vi "Primer programa1.vi"() -> ()   [LabVIEW 2020]
panel:
  out "String":string
  out "Resultado":dbl
  in  "y":dbl
  in  "x":dbl
  in  "Opcion":string(combo)="Suma"
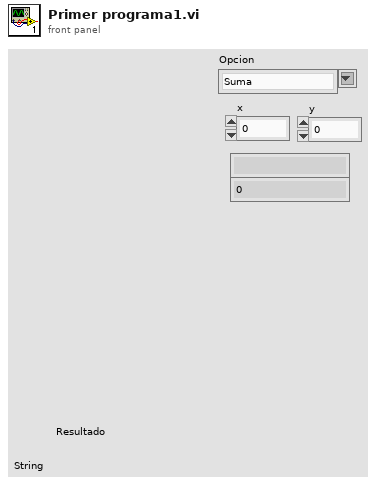
[diagram p1: front panel]
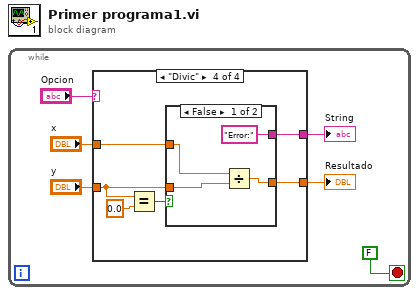
[diagram p0: block diagram]
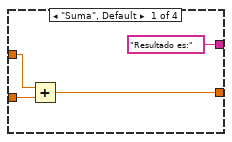
[diagram p2: hidden frame]
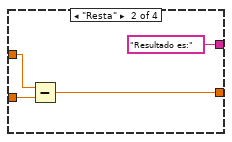
[diagram p3: hidden frame]
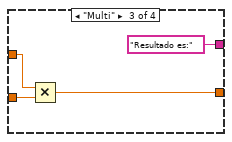
[diagram p4: hidden frame]
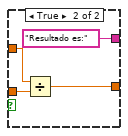
[diagram p5: hidden frame]
diagram:
  n1 = while {
    stop <- FALSE stop-if-true
    n2 = case shown="\"Divic\"" "Opcion" {
      tunnel: "x" -> [w10 w14 w18 w22]
      tunnel: "y" -> [w9 w13 w17 w21]
      tunnel: [w8 w12 w15 w20] -> w2
      tunnel: ["Resultado es:" ("String") "Resultado es:" ("String") "Resultado es:" ("String") w19] -> w1
      frame "Suma", Default {
        n3 = Add(x=w10, y=w9) -> (x+y=w8:dbl)
      }
      frame "Resta" {
        n4 = Subtract(x=w14, y=w13) -> (x-y=w12:dbl)
      }
      frame "Multi" {
        n5 = Multiply(x=w18, y=w17) -> (x*y=w15:dbl)
      }
      frame "Divic" {
        n6 = Equal?(x=w21, y=0.0) -> (x = y?=w23:bool)
        n7 = case shown="False" w23 {
          tunnel: w22 -> [w27 w32]
          tunnel: w21 -> [w28 w31]
          tunnel: [w26 w30] -> w20
          tunnel: ["Error:" ("String") "Resultado es:" ("String")] -> w19
          frame False {
            n8 = Divide(x=w27, y=w28) -> (x/y=w26:dbl)
          }
          frame True {
            n9 = Divide(x=w32, y=w31) -> (x/y=w30:dbl)
          }
        }
      }
    }
    "Resultado" <- w2
    "String" <- w1
  }
